vi "Flow Probe.vi"(11 "TLB` Template.lvlib:TLB' Template.lvclass":refnum<class "{TMPL} TLB`.lvclass">) -> (2 "Value String":string, 3 "Boolean":bool)   [LabVIEW 2026, in "Synchronize AWS S3 Content.lvlib" / "{TMPL} TLB`.lvclass"]
uses:
  {TMPL} TLB`.lvclass
  {TMPL} TLB`.lvclass/{TMPL} TLB`.ctl
  Application Components/Trigger API/System Trigger.ctl
  Application Components/Trigger API/{TMPL} Trigger API.lvlib
  State Machine/State.ctl
panel:
  out "history":T3(array[cluster])
  in  "length":i32=20
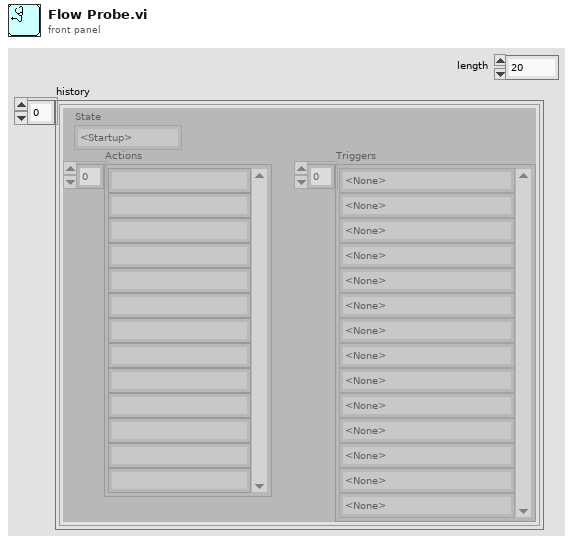
[diagram p1: front panel]
types:
  T1 = typedef "Synchronize AWS S3 Content.lvlib/{TMPL} TLB`.lvclass/State.ctl" = enum16{"<Startup>", "Idle", "<Shutdown>", "<Error>"}
  T2 = typedef "Synchronize AWS S3 Content.lvlib/{TMPL} Trigger API.lvlib/System Trigger.ctl" = enum16{"<None>", "Connect", "Start Acquisition", "Stop Acquisition", "Disconnect", "<Return to Safe State Actions>", "<Cache User Parameters>", "<Close Application>", "<Error>"}
  T3 = cluster{"State":T1, "Actions":string[], "Triggers":T2[]}[]
  T4 = typedef "Synchronize AWS S3 Content.lvlib/{TMPL} Trigger API.lvlib/System Trigger Element.ctl" = cluster{"System Trigger":T2, "Trigger Data":variant}
  T5 = typedef "Synchronize AWS S3 Content.lvlib/Actions.lvlib/System Action Element.ctl" = cluster{"action":string, "data":string}
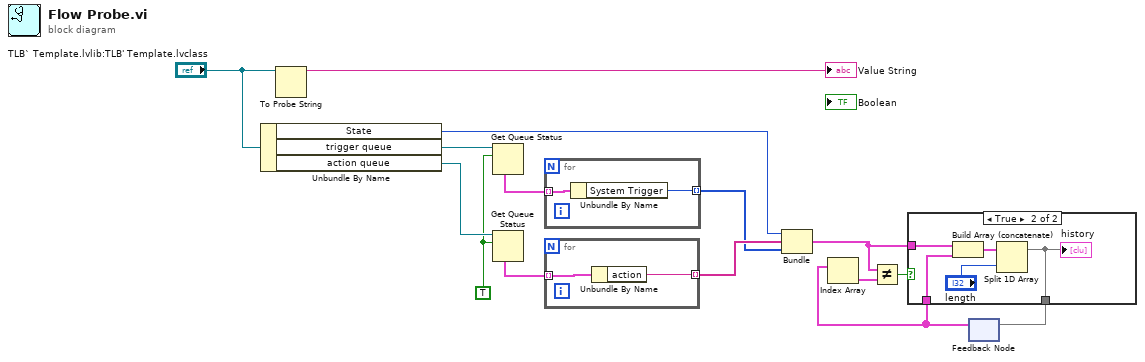
[diagram p0: block diagram]
diagram:
  w11 = TRUE ("return elements? (F)")
  n1 = Unbundle By Name("TLB` Template.lvlib:TLB' Template.lvclass") -> ("State"=w1:T1, "trigger queue"=w13:refnum<queue>, "action queue"=w12:refnum<queue>)
  n2 = To Probe String(7:"TLB` Template.lvlib:TLB' Template.lvclass") -> (3:→"Value String":string)  [unwired: 2 in, 1 out]
  n3 = Get Queue Status(queue=w13, return elements? (F)=w11) -> (elements=w10:T4[])  [unwired: 1 in, 7 out]
  n4 = Get Queue Status(queue=w12, return elements? (F)=w11) -> (elements=w9:T5[])  [unwired: 1 in, 7 out]
  n5 = for {
    tunnel: w10 -> [w17] mode=indexing
    tunnel: [w16] -> w7 mode=indexing
    n6 = Unbundle By Name(w17) -> ("System Trigger"=w16:T2)
  }
  n7 = for {
    tunnel: w9 -> [w19] mode=indexing
    tunnel: [w18] -> w8 mode=indexing
    n8 = Unbundle By Name(w19) -> ("action"=w18:string)
  }
  n9 = Bundle("State"=w1, w8, w7) -> (w3:cluster{"State":T1, string[], T2[]})  [unwired: 1 in]
  n10 = feedback #1() -> (w5:cluster{"State":T1, string[], T2[]}[])  [unwired: 1 in]
  n11 = Index Array(array=w5) -> (element=w4:cluster{"State":T1, string[], T2[]})  [unwired: 1 in]
  n12 = Not Equal?(x=w3, y=w4) -> (x != y?=w2:bool)
  n13 = case shown="True" w2 {
    tunnel: [w20 w23] -> w6
    tunnel: w5 -> [w20 w22]
    tunnel: w3 -> [_ w21]
    frame False {
    }
    frame True {
      n14 = Build Array (concatenate)(w21, w22) -> (w25:cluster{"State":T1, string[], T2[]}[])
      n15 = Split 1D Array(array=w25, index="length") -> (first subarray=w23:cluster{"State":T1, string[], T2[]}[])  [unwired: 1 out]
      "history" <- w23
    }
  }
  n16 = feedback-in #1(w6) -> ()
